vi "Calibration to String.vi"(10 "fs cal array":dbl[][](array[numeric]), 11 "fs cal results":dbl[][](array[numeric])) -> (3 "cal string":string)   [LabVIEW 2020]
uses:
  <vilib>/Analysis/baseanly.llb/Mean (DBL).vi
  <vilib>/Analysis/NI_AALBase.lvlib
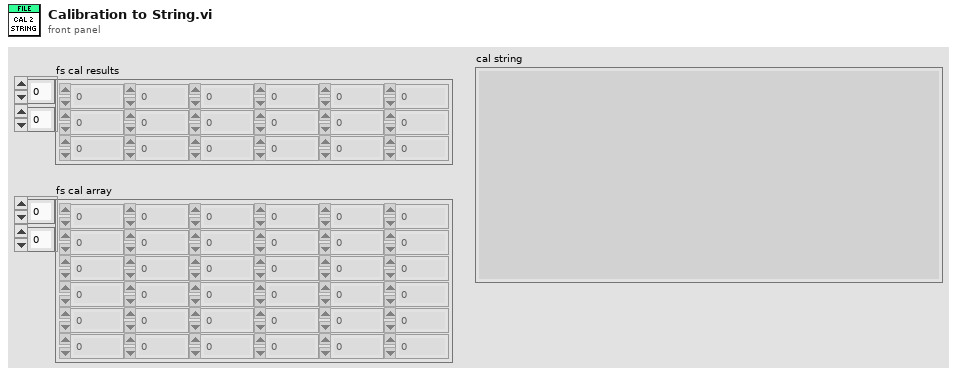
[diagram p1: front panel]
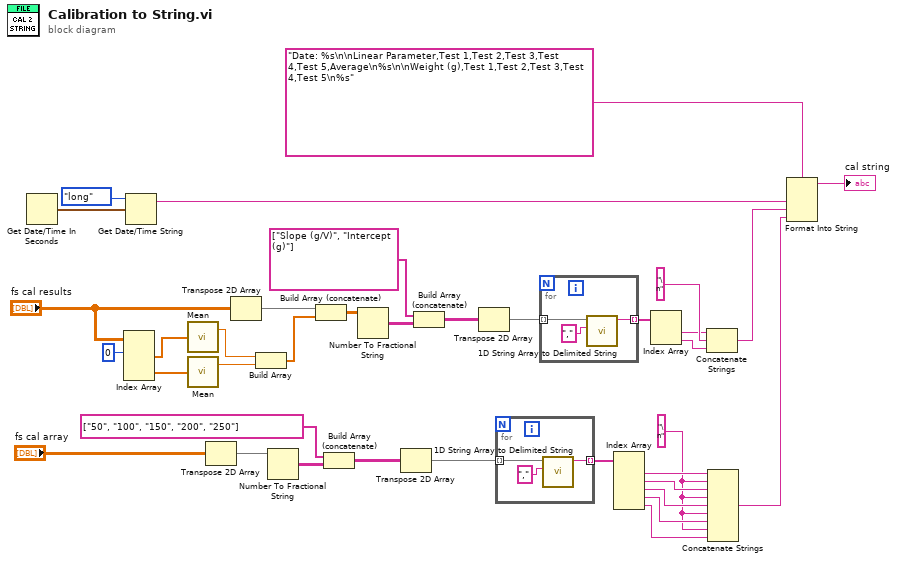
[diagram p0: block diagram]
diagram:
  w13 = "\n" ("string")
  n1 = Get Date/Time In Seconds() -> (seconds since 1Jan1904=w21:timestamp)
  n2 = Index Array(array="fs cal results", index (row) #1=0 ("index (row)")) -> (element #1=w36:dbl[], element #2=w35:dbl[])  [unwired: 3 in]
  n3 = Get Date/Time String(date format (0)=enum16{"short", "long", "abbreviated"}."long", seconds (now)=w21) -> (date string=w23:string)  [unwired: 1 in, 1 out]
  n4 = call-poly <vilib>:"Mean.vi"("X"=w36) -> ("mean"=w34:dbl)  [unwired: 1 out]
  n5 = call-poly <vilib>:"Mean.vi"("X"=w35) -> ("mean"=w33:dbl)  [unwired: 1 out]
  n6 = Transpose 2D Array(2D array="fs cal array") -> (transposed array=w3:dbl[][])
  n7 = Transpose 2D Array(2D array="fs cal results") -> (transposed array=w7:dbl[][])
  n8 = Build Array(w34, w33) -> (w32:dbl[])
  n9 = Number To Fractional String(number=w3) -> (F-format string=w19:string[][])  [unwired: 3 in]
  n10 = Build Array (concatenate)(w7, w32) -> (w31:dbl[][])
  n11 = Build Array (concatenate)(string[] ["50", "100", "150", "200", "250"], w19) -> (w2:string[][])
  n12 = Number To Fractional String(number=w31) -> (F-format string=w29:string[][])  [unwired: 3 in]
  n13 = Transpose 2D Array(2D array=w2) -> (transposed array=w1:string[][])
  n14 = Build Array (concatenate)(string[] ["Slope (g/V)", "Intercept (g)"], w29) -> (w6:string[][])
  n15 = Transpose 2D Array(2D array=w6) -> (transposed array=w5:string[][])
  n16 = for {
    tunnel: [w39] -> w18 mode=indexing
    tunnel: w1 -> [w38] mode=indexing
    n17 = call <vilib>:"1D String Array to Delimited String.vi"("delimiter"=",", "string array"=w38) -> ("delimited string"=w39:string)  [unwired: 9 in]
  }
  n18 = for {
    tunnel: w5 -> [w43] mode=indexing
    tunnel: [w41] -> w28 mode=indexing
    n19 = call <vilib>:"1D String Array to Delimited String.vi"("delimiter"=",", "string array"=w43) -> ("delimited string"=w41:string)  [unwired: 9 in]
  }
  n20 = Index Array(array=w18) -> (element #1=w17:string, element #2=w16:string, element #3=w15:string, element #4=w14:string, element #5=w12:string)  [unwired: 5 in]
  n21 = Index Array(array=w28) -> (element #1=w25:string, element #2=w27:string)  [unwired: 2 in]
  n22 = Concatenate Strings(w25, "\n" ("string"), w27) -> (w11:string)
  n23 = Concatenate Strings(w17, w13, w16, w13, w15, w13, w14, w13, w12) -> (w10:string)
  n24 = Format Into String(format string="Date: %s\n\nLinear Parameter,Test 1,Test 2,Test 3,Test 4,Test 5,Average\n%s\n\nWeight (g),Test 1,Test 2,Test 3,Test 4,Test 5\n%s", w23, w11, w10) -> (resulting string=→"cal string":string)  [unwired: 2 in, 1 out]
